vi "ErrorLog (SubVI).vi"(8 "Application ref in":refnum<vi>, 10 "Status":string, 11 "Byte Stream File in":refnum<file>) -> (0 "Application ref out":refnum<vi>)   [LabVIEW 2014]
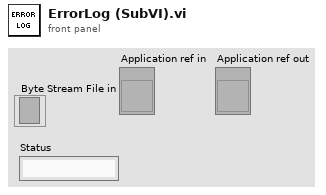
[diagram p1: front panel]
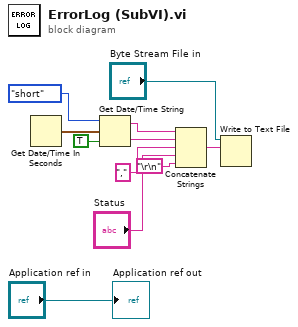
[diagram p0: block diagram]
diagram:
  n1 = Get Date/Time In Seconds() -> (seconds since 1Jan1904=w6:timestamp)
  n2 = Get Date/Time String(date format (0)=enum16{"short", "long", "abbreviated"}."short", seconds (now)=w6, want seconds? (F)=TRUE) -> (date string=w3:string, time string=w4:string)
  n3 = Concatenate Strings(w3, w4, "," ("string"), "Status", "\r\n") -> (w9:string)
  n4 = Write to Text File(file (use dialog)="Byte Stream File in", text=w9) -> ()  [unwired: 2 in, 3 out]
  "Application ref out" <- "Application ref in"
